vi "Get value by Variant.vi"(8 "error in (no error)":errorcluster, 11 "Ctrl Refnum Column in":refnum<class "Ctrl Refnum Column.lvclass">) -> (0 "error out":errorcluster, 2 "Variant":variant, 3 "Ctrl Refnum Column out":refnum<class "Ctrl Refnum Column.lvclass">)   [LabVIEW 2020, in "Basic Fields.lvlib" / "Ctrl Refnum Column.lvclass"]
uses:
  Ctrl Refnum Column.lvclass
  Ctrl Refnum Column.lvclass/Ctrl Refnum Column.ctl
  Basic Columns/Basic Columns/Column Class/Column Parent.lvclass
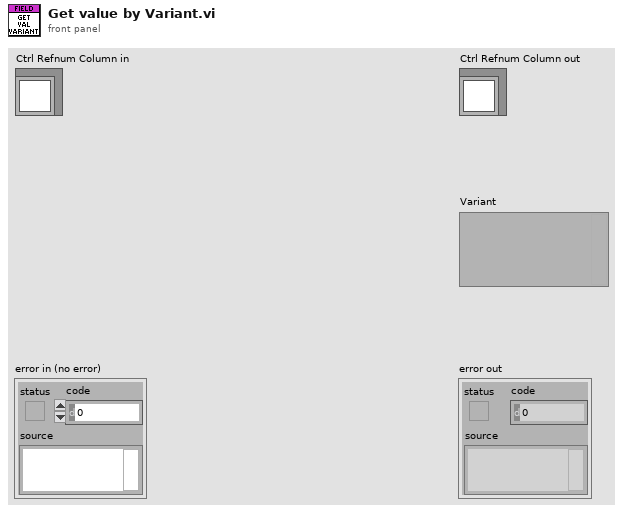
[diagram p1: front panel]
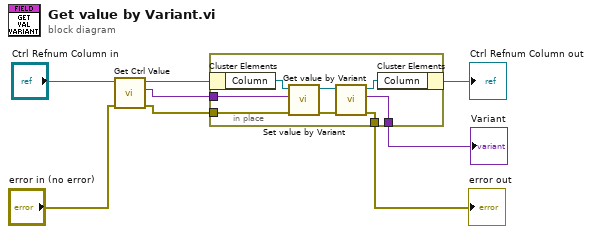
[diagram p0: block diagram]
diagram:
  n1 = call-dynamic "Get Ctrl Value.vi"("error in (no error)"="error in (no error)", "Ctrl Refnum Column in"="Ctrl Refnum Column in") -> ("error out"=w8:errorcluster, "Ctrl Value"=w7:variant, "Ctrl Refnum Column out"=w6:refnum<class "Ctrl Refnum Column.lvclass">)  [unwired: 7 in]
  n2 = in-place {
    in-place-border: w7 -> [w15]
    in-place-border: w8 -> [w14]
    in-place-border: [w10] -> w2
    in-place-border: [w9] -> w1
    n3 = in-place-cluster #1(w6) -> ("Column"=w16:refnum<class "Column Parent.lvclass">)
    n4 = call-dynamic "Set value by Variant.vi"("error in (no error)"=w14, "Variant"=w15, "Column in"=w16) -> ("error out"=w11:errorcluster, "Column out"=w13:refnum<class "Column Parent.lvclass">)  [unwired: 7 in]
    n5 = call-dynamic "Get value by Variant.vi"("error in (no error)"=w11, "Column Parent in"=w13) -> ("error out"=w9:errorcluster, "Variant"=w10:variant, "Column Parent out"=w12:refnum<class "Column Parent.lvclass">)  [unwired: 7 in]
    n6 = in-place-cluster #1("Column"=w12) -> (→"Ctrl Refnum Column out":refnum<class "Ctrl Refnum Column.lvclass">)
  }
  "error out" <- w1
  "Variant" <- w2
